vi "ThingWorxmyRio.vi"(0 "End Session":bool) -> (1 "Properties from ThingWorx":string[][](array[string])=[["Button", "true"], ["Button2", "true"], ["description", ""], ["isConnected", "false"], ["lastConnection", "1970-01-01T00:00:00.000Z"], ["name", "GenericEdge"], ["Photocell", "200.0"], ["Potentiometer", "234.0"], ["tags", "GenericRemoteEdge:Example"], ["Temperature", "0.242"], ["thingTemplate", "GenericThingTemplate"]])   [LabVIEW 2015]
uses:
  <vilib>/myRIO/Instrument Drivers/Onboard IO/AI/typedefs/AI Reference.ctl
  <vilib>/myRIO/Common/Instrument Driver Framework/Utilities/typedefs/myRIO Generic Hardware Reference.ctl
  <vilib>/myRIO/Common/Instrument Driver Framework/Utilities/typedefs/Hardware Version Enum.ctl
  <vilib>/myRIO/Common/Instrument Driver Framework/Utilities/typedefs/myRIO v1.0 Reference.ctl
  <vilib>/myRIO/Common/Instrument Driver Framework/Utilities/typedefs/Generic FPGA Reference.ctl
  <vilib>/myRIO/Common/Instrument Driver Framework/myRIO v1.0/AI/typedefs/AI Channels List.ctl
  <vilib>/myRIO/Common/Instrument Driver Framework/myRIO v1.0/AI/typedefs/AI Channels Enum.ctl
  <vilib>/myRIO/Common/Instrument Driver Framework/Utilities/typedefs/Analog Scaling Constants List.ctl
  <vilib>/myRIO/Common/Instrument Driver Framework/Utilities/typedefs/Analog Scaling Constants.ctl
  <vilib>/userdefined/High Color/nirio_resource_hc.ctl
  <vilib>/myRIO/Instrument Drivers/Onboard IO/DIO/typedefs/DIO Reference.ctl
  <vilib>/myRIO/Common/Instrument Driver Framework/myRIO v1.0/DIO/typedefs/DIO Channels List.ctl
  <vilib>/myRIO/Common/Instrument Driver Framework/myRIO v1.0/DIO/typedefs/DIO Channels Enum.ctl
  <vilib>/myRIO/Common/Instrument Driver Framework/Utilities/vis/Is FPGA Ref Available.vi
  <vilib>/myRIO/Common/Instrument Driver Framework/myRIO v1.0/AI/vis/myRIO v1.1 Open AI.vi
  <vilib>/myRIO/Instrument Drivers/Onboard IO/AI/vis/Read.vi
  <vilib>/myRIO/Common/Instrument Driver Framework/myRIO v1.0/DIO/vis/myRIO v1.1 Open DIO.vi
  <vilib>/myRIO/Instrument Drivers/Onboard IO/DIO/vis/Read.vi
  <vilib>/myRIO/Common/Instrument Driver Framework/Utilities/vis/Validate Channels.vi
  <vilib>/myRIO/Common/Instrument Driver Framework/myRIO v1.0/AI/vis/myRIO v1.0 Reserve AI.vi
  <vilib>/myRIO/Common/Instrument Driver Framework/myRIO v1.0/DIO/vis/myRIO v1.0 Reserve DIO.vi
  <vilib>/myRIO/Common/Instrument Driver Framework/myRIO v1.0/AI/vis/myRIO v1.0 Build MUX Configuration AI.vi
  <vilib>/myRIO/Common/Instrument Driver Framework/myRIO v1.0/Resource Manager/vis/myRIO v1.0 Reserve Channel List.vi
  <vilib>/myRIO/Common/Instrument Driver Framework/myRIO v1.0/DIO/vis/myRIO v1.0 Build MUX Configuration DIO.vi
  <vilib>/myRIO/Common/Instrument Driver Framework/myRIO v1.0/Resource Manager/vis/myRIO v1.0 Reserve Channel.vi
  <vilib>/myRIO/Common/Instrument Driver Framework/myRIO v1.0/Resource Manager/vis/myRIO v1.0 Unreserve Channel.vi
  <vilib>/myRIO/Common/Instrument Driver Framework/myRIO v1.0/Resource Manager/vis/myRIO v1.0 Create Configuration List.vi
  <vilib>/myRIO/Common/Instrument Driver Framework/myRIO v1.0/Resource Manager/vis/myRIO v1.0 Build Mutex Name.vi
  <vilib>/Utility/VariantDataType/GetNumericInfo.vi
  <vilib>/Utility/error.llb/Error Cluster From Error Code.vi
  <vilib>/myRIO/Common/Instrument Driver Framework/myRIO v1.0/myRIO v1.1 Open.vi
  <vilib>/myRIO/Common/Instrument Driver Framework/myRIO v1.0/AI/vis/myRIO v1.0 Get Scaling Constants AI.vi
  <vilib>/myRIO/Common/Instrument Driver Framework/Utilities/vis/IO Manager.vi
  <vilib>/myRIO/Common/Instrument Driver Framework/Utilities/vis/Configuration Manager.vi
  <vilib>/myRIO/Common/Instrument Driver Framework/myRIO v1.0/myRIO v1.0 Close.vi
  <vilib>/myRIO/Common/Instrument Driver Framework/myRIO v1.0/AI/vis/myRIO v1.0 Read AI.vi
  <vilib>/myRIO/Common/Instrument Driver Framework/myRIO v1.0/Resource Manager/vis/myRIO v1.0 Configure IO.vi
  <vilib>/myRIO/Common/Instrument Driver Framework/myRIO v1.0/DIO/vis/myRIO v1.0 Read DIO.vi
  <vilib>/myRIO/Express VI/Onboard IO/AI/AI Express VI.xnode
  <vilib>/myRIO/Instrument Drivers/Onboard IO/AI/vis/myRIO AI Open.xnode
  <vilib>/myRIO/Express VI/Onboard IO/DI/DI Express VI.xnode
  <vilib>/myRIO/Instrument Drivers/Onboard IO/DIO/vis/myRIO DIO Open.xnode
  <vilib>/myRIO/Express VI/Onboard Devices/Button/Button Express VI.xnode
  <vilib>/httpClient/LabVIEWHTTPClient.lvlib
  <vilib>/myRIO/Instrument Drivers/Onboard IO/AI/AI.lvlib
  <vilib>/myRIO/Instrument Drivers/Onboard IO/DIO/DIO.lvlib
panel:
  in  "Properties in Service":string[](array[string])=["Button", "Potentiometer", "Temperature", "Photocell", "Button2"]
  in  "Input Info":T1={"ThingWorx Server Address"="52.202.159.58", "Port"="80", "Thing Name"="GenericEdge", "Application Key"="0aae8b5f-871a-4973-bdf2-199fabb27dcb", "Service Name"="UpdateValues"}
  out "Photocell":dbl(knob) scale=0.0..5.0
  out "Potentiometer":dbl(knob) scale=0.0..5.0
  out "Button":bool
  out "Thermometer":dbl(slide) scale=0.0..100.0
  out "Button2":bool
  out "error out":errorcluster
  # "*Make sure you download the \"HTTP Client with SSL Support\" library on to your myRio before running this VI (and possibly \"I/O Variable Remote Config. Web Service,\" \n\"NI Application Web Server,\" \"Variable Client Support for LabVIEW RT,\" and \"WebDAV Client with SSL Support.\""
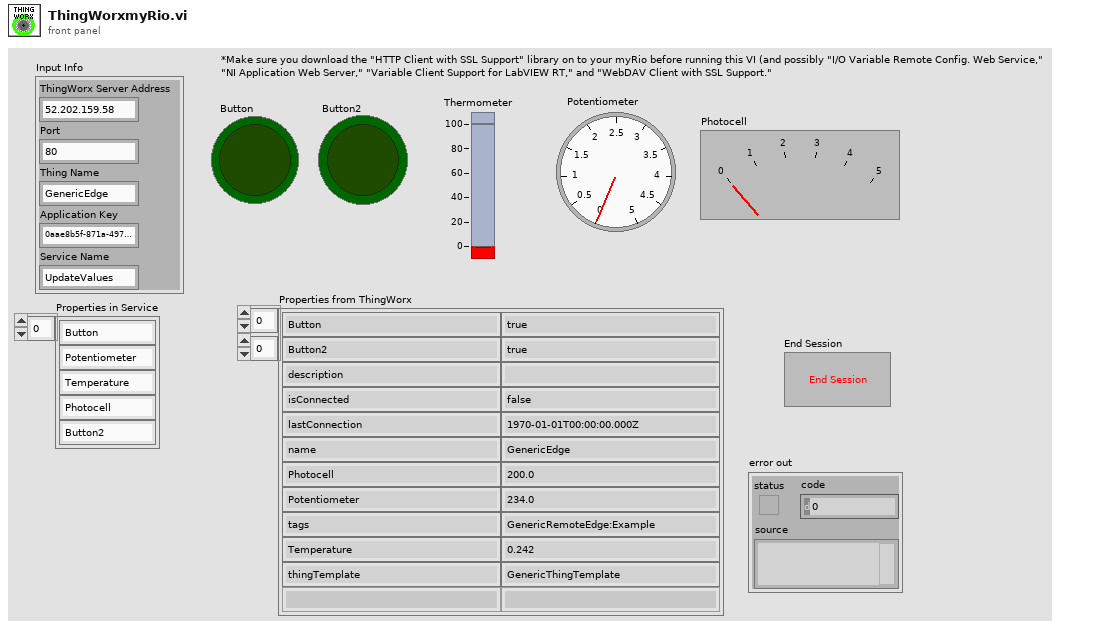
[diagram p1: front panel]
types:
  T1 = cluster{"ThingWorx Server Address":string, "Port":string, "Thing Name":string, "Application Key":string, "Service Name":string}
  T2 = typedef "LabVIEWHTTPClient.lvlib/ClientHandle.ctl" = refnum<k1>
  T3 = cluster{"client handle":T2, "Url Beginning":string, "App Key":string, "Service Name":string, "Properties":string[]}
  T4 = typedef "DIO.lvlib/DIO Reference.ctl" = cluster{"myRIO Reference":T5, "DIO Channels List":T9}
  T5 = typedef "myRIO Generic Hardware Reference.ctl" = cluster{"myRIO Model":T6, "myRIO Hardware Reference":T7}
  T6 = typedef "Hardware Version Enum.ctl" = enum16{"Unknown", "myRIO-1900", "myRIO-1950", "roboRIO"}
  T7 = typedef "myRIO v1.0 Reference.ctl" = cluster{"Generic FPGA Reference":T8, "Allow multiple opens":bool}
  T8 = typedef "Generic FPGA Reference.ctl" = refnum<k20>
  T9 = typedef "DIO Channels List.ctl" = T10[]
  T10 = typedef "DIO Channels Enum.ctl" = enum16{"Not Connected", "C/DIO0", "C/DIO1", "C/DIO2", "C/DIO3", "C/DIO4", "C/DIO5", "C/DIO6", "C/DIO7", "A/DIO0", "A/DIO1", "A/DIO2", "A/DIO3", "A/DIO4", "A/DIO5", "A/DIO6", "A/DIO7", "A/DIO8", "A/DIO9", "A/DIO10", "A/DIO11", "A/DIO12", "A/DIO13", "A/DIO14", "A/DIO15", "B/DIO0", "B/DIO1", "B/DIO2", "B/DIO3", "B/DIO4", "B/DIO5", "B/DIO6", "B/DIO7", "B/DIO8", "B/DIO9", "B/DIO10", "B/DIO11", "B/DIO12", "B/DIO13", "B/DIO14", "B/DIO15", "LED0", "LED1", "LED2", "LED3", "Button0", "DIO/DIO0", "DIO/DIO1", "DIO/DIO2", "DIO/DIO3", "DIO/DIO4", "DIO/DIO5", "DIO/DIO6", "DIO/DIO7", "DIO/DIO8", "DIO/DIO9", "SPI/CS0", "SPI/CS1", "SPI/CS2", "SPI/CS3", "LED RADIO (Green)", "LED RADIO (Red)", "LED COMM (Green)", "LED COMM (Red)", "LED MODE (Green)", "LED MODE (Red)"}
  T11 = typedef "nirio_resource_hc.ctl" = tag
  T12 = typedef "AI.lvlib/AI Reference.ctl" = cluster{"myRIO Reference":T5, "AI Channels List":T13, "AI Scaling Constants List":T15}
  T13 = typedef "AI Channels List.ctl" = T14[]
  T14 = typedef "AI Channels Enum.ctl" = enum16{"Not Connected", "AudioIn/Left", "AudioIn/Right", "C/AI0", "C/AI1", "A/AI0", "A/AI1", "A/AI2", "A/AI3", "B/AI0", "B/AI1", "B/AI2", "B/AI3", "AI/AI0", "AI/AI1", "AI/AI2", "AI/AI3"}
  T15 = typedef "Analog Scaling Constants List.ctl" = T16[]
  T16 = typedef "Analog Scaling Constants.ctl" = cluster{"LSB Weight (Volts)":dbl, "Offset (Volts)":dbl, "Signed?":bool}
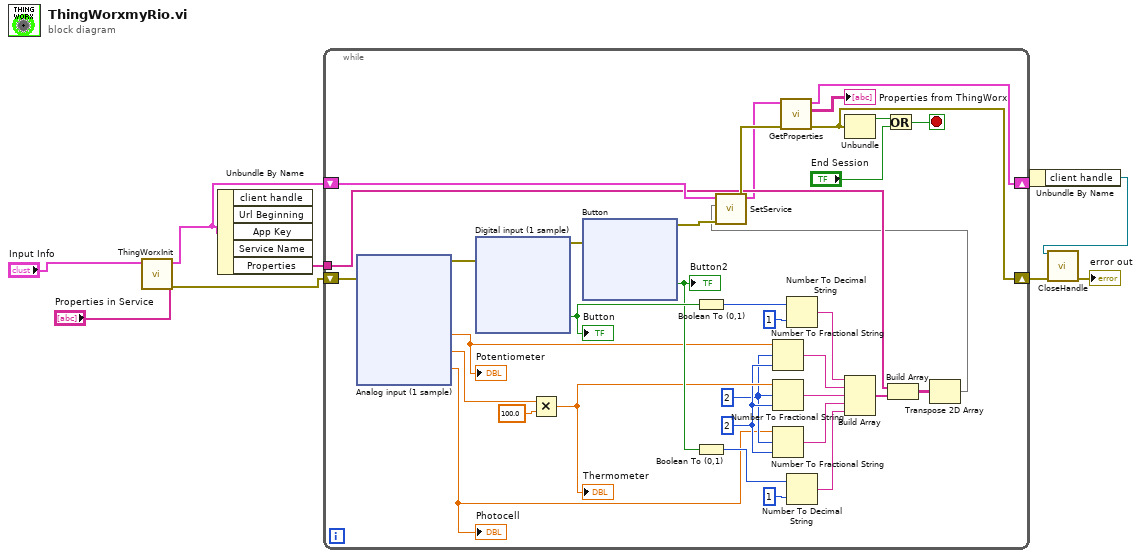
[diagram p0: block diagram]
diagram:
  n1 = call "ThingWorxInit.vi"("Properties"="Properties in Service", "Input Info"="Input Info") -> ("error out"=w1:errorcluster, "Thing Info Out"=w2:T3)  [unwired: 8 in]
  n2 = Unbundle By Name(w2) -> ("Properties"=w6:string[])  [unwired: 4 out]
  n3 = while {
    shift-right: [w39] -> w9
    shift-left: w1 -> [w30]
    shift-right: [w11] -> w5
    shift-left: w2 -> [w14]
    tunnel: w6 -> [w13]
    stop <- w44 stop-if-true
    w18 = i16 2 ("precision (6)")
    w17 = i16 2 ("width (-)")
    n4 = xnode "Analog input (1 sample)"("error in (no error)"=w30) -> ("B/AI0 (Pin 3)"=w19:dbl, "B/AI1 (Pin 5)"=w23:dbl, "B/AI2 (Pin 7)"=w15:dbl, "error out"=w29:errorcluster)
    "Potentiometer" <- w19
    "Photocell" <- w15
    n5 = xnode "Digital input (1 sample)"("error in (no error)"=w29) -> ("B/DIO0 (Pin 11)"=w28:bool, "error out"=w27:errorcluster)
    "Button" <- w28
    n6 = Multiply(x=w23, y=100.0) -> (x*y=w21:dbl)
    "Thermometer" <- w21
    n7 = xnode "Button"("error in (no error)"=w27) -> ("Value"=w25:bool, "error out"=w26:errorcluster)
    "Button2" <- w25
    n8 = Boolean To (0,1)(Boolean=w28) -> (0, 1=w35:i16)
    n9 = Boolean To (0,1)(Boolean=w25) -> (0, 1=w37:i16)
    n10 = Number To Fractional String(number=w19, width (-)=w17, precision (6)=w18) -> (F-format string=w20:string)  [unwired: 1 in]
    n11 = Number To Fractional String(number=w21, width (-)=w17, precision (6)=w18) -> (F-format string=w22:string)  [unwired: 1 in]
    n12 = Number To Fractional String(number=w15, width (-)=w17, precision (6)=w18) -> (F-format string=w16:string)  [unwired: 1 in]
    n13 = Number To Decimal String(number=w35, width (-)=i16 1) -> (decimal integer string=w34:string)
    n14 = Number To Decimal String(number=w37, width (-)=i16 1) -> (decimal integer string=w33:string)
    n15 = Build Array(w34, w20, w22, w16, w33) -> (w31:string[])
    n16 = Build Array(w13, w31) -> (w32:string[][])
    n17 = Transpose 2D Array(2D array=w32) -> (transposed array=w12:string[][])
    n18 = call "SetService.vi"("error in"=w26, "Properties"=w12, "Thing Info In"=w14) -> ("error out"=w40:errorcluster, "Thing Info Out"=w10:T3)  [unwired: 7 in]
    n19 = call "GetProperties.vi"("error in (no error)"=w40, "Thing Info In"=w10) -> ("error out"=w39:errorcluster, "Array"=→"Properties from ThingWorx":string[][], "Thing Info Out"=w11:T3)  [unwired: 7 in]
    n20 = Unbundle(w39) -> ("status"=w42:bool)  [unwired: 2 out]
    n21 = Or(x=w42, y="End Session") -> (x .or. y?=w44:bool)
  }
  n22 = Unbundle By Name(w5) -> ("client handle"=w4:T2)
  n23 = call <vilib>:"CloseHandle.vi"("client handle"=w4, "error in (no error)"=w9) -> ("error out"=→"error out":errorcluster)  [unwired: 13 in]
